vi "02guarda_archivo.vi"(0 "file path nvo":path, 1 "Mediciones":T1, 2 "Mapas Eeprom":T2(array[cluster]), 4 "Equipo nº":i32=30 caption="Eq. nº" min=25 max=100 step=5) -> (5 "error out":errorcluster)   [LabVIEW 2010]
uses:
  <vilib>/Utility/file.llb/Write To Spreadsheet File (string).vi
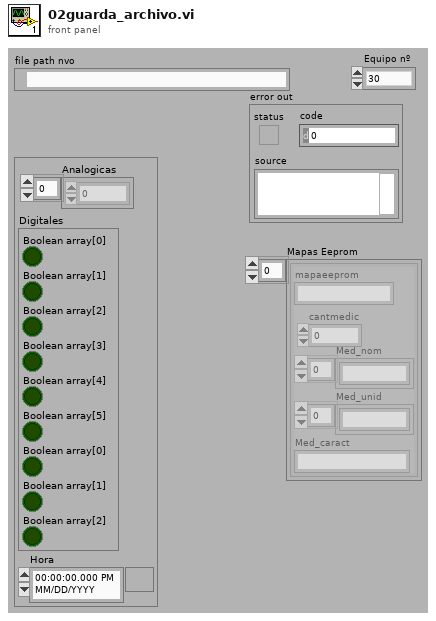
[diagram p1: front panel]
types:
  T1 = cluster{"Analogicas":dbl[], "Digitales":cluster{"Boolean array[0]":bool, "Boolean array[1]":bool, "Boolean array[2]":bool, "Boolean array[3]":bool, "Boolean array[4]":bool, "Boolean array[5]":bool, "Boolean array[0]":bool, "Boolean array[1]":bool, "Boolean array[2]":bool}, "Hora":timestamp}
  T2 = cluster{"mapaeeprom":string, "cantmedic":u8, "Med_nom":string[], "Med_unid":string[], "Med_caract":string}[]
  T3 = enum16{"open", "replace", "create", "open or create", "replace or create", "replace or create with confirmation"}
  T4 = cluster{"Boolean array[0]":bool, "Boolean array[1]":bool, "Boolean array[2]":bool, "Boolean array[3]":bool, "Boolean array[4]":bool, "Boolean array[5]":bool, "Boolean array[0]":bool, "Boolean array[1]":bool, "Boolean array[2]":bool}
  T5 = cluster{"mapaeeprom":string, "cantmedic":u8, "Med_nom":string[], "Med_unid":string[], "Med_caract":string}
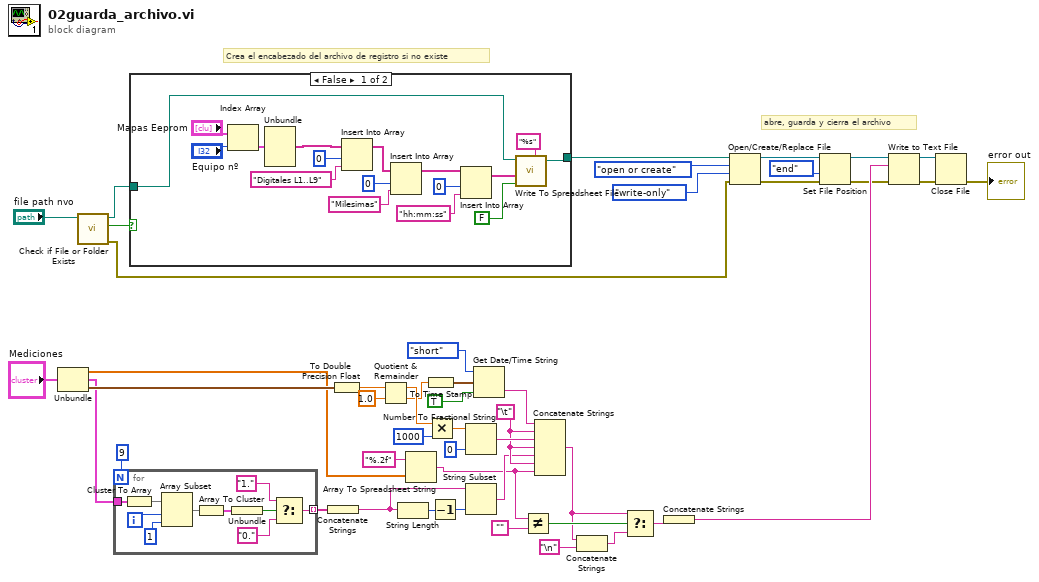
[diagram p0: block diagram]
diagram:
  w26 = "\t"
  # "abre, guarda y cierra el archivo"
  # "Crea el encabezado del archivo de registro si no existe"
  n1 = Unbundle("Mediciones") -> ("Analogicas"=w17:dbl[], "Digitales"=w18:T4, "Hora"=w19:timestamp)
  n2 = call <vilib>:"Check if File or Folder Exists.vi"("path"="file path nvo") -> ("error out"=w1:errorcluster, "file or folder exists?"=w4:bool, "dup path"=w3:path)  [unwired: 8 in]
  n3 = for {
    N: 9 -> [_]
    tunnel: w18 -> [w57]
    tunnel: [w50] -> w24 mode=indexing
    i -> [w52]
    n4 = Cluster To Array(cluster=w57) -> (array=w56:bool[])
    n5 = Array Subset(array=w56, index=w52, length=1) -> (w55:bool[])
    n6 = Array To Cluster(array=w55) -> (cluster=w54:cluster{"[0]":bool})
    n7 = Unbundle(w54) -> ("[0]"=w51:bool)
    n8 = Select(t="1.", s=w51, f="0.") -> (s? t:f=w50:string)
  }
  n9 = case shown="False" w4 {
    tunnel: w3 -> [w63 w75]
    tunnel: [w62 w75] -> w7
    frame False {
      n10 = Index Array(array="Mapas Eeprom", index="Equipo nº") -> (element=w61:T5)
      n11 = Unbundle(w61) -> ("Med_nom"=w58:string[])  [unwired: 4 out]
      n12 = Insert Into Array(array=w58, index=0, new element="Digitales L1..L9" ("new element/subarray")) -> (w71:string[])
      n13 = Insert Into Array(array=w71, index=0, new element="Milesimas" ("new element/subarray")) -> (w69:string[])
      n14 = Insert Into Array(array=w69, index=0, new element="hh:mm:ss" ("new element/subarray")) -> (w68:string[])
      n15 = call-poly <vilib>:"Write To Spreadsheet File.vi"("format (%s)"="%s", "append to file? (new file:F)"=FALSE, "1D data"=w68, "file path (dialog if empty)"=w63) -> ("new file path (Not A Path if cancelled)"=w62:path)  [unwired: 2 in, 2 out]
    }
    frame True {
    }
  }
  n16 = Concatenate Strings(w24) -> (w20:string)
  n17 = To Double Precision Float(number=w19) -> (double precision float=w23:dbl)
  n18 = Quotient & Remainder(x=w23, y=1.0) -> (x-y*floor(x/y)=w32:dbl, floor(x/y)=w27:dbl)
  n19 = String Length(string=w20) -> (length=w22:i32)
  n20 = Array To Spreadsheet String(array=w17, 3:"%.2f" ("format string")) -> (spreadsheet string=w11:string)  [unwired: 1 out]
  n21 = To Time Stamp(1:w27) -> (0:w30:timestamp)
  n22 = Multiply(x=w32, y=1000 ("index")) -> (x*y=w36:dbl)
  n23 = Decrement(x=w22) -> (x-1=w21:i32)
  n24 = Number To Fractional String(number=w36, precision (6)=i16 0) -> (F-format string=w35:string)  [unwired: 2 out]
  n25 = String Subset(string=w20, length (rest)=w21) -> (substring=w16:string)  [unwired: 1 out]
  n26 = Get Date/Time String(date format (0)=enum16{"short", "long", "abbreviated"}."short", seconds (now)=w30, want seconds? (F)=TRUE) -> (time string=w34:string)  [unwired: 1 out]
  n27 = Not Equal?(x=w11, y="") -> (x != y?=w15:bool)
  n28 = Concatenate Strings(w34, w26, w35, w26, w16, w26, w11) -> (w14:string)
  n29 = Concatenate Strings(w14, "\n") -> (w13:string)
  n30 = Select(t=w14, s=w15, f=w13) -> (s? t:f=w42:string)
  n31 = Concatenate Strings(w42) -> (w41:string)
  n32 = Open/Create/Replace File(file path (use dialog)=w7, error in=w1, operation (0:open)=T3."open or create", access (0:read/write)=enum16{"read/write", "read-only", "write-only"}."write-only") -> (refnum out=w47:refnum<file>, error out=w39:errorcluster)  [unwired: 3 out]
  n33 = Set File Position(refnum=w47, from (0:start)=enum16{"start", "end", "current"}."end", error in=w39) -> (refnum out=w43:refnum<file>, error out=w8:errorcluster)  [unwired: 1 out]
  n34 = Write to Text File(file (use dialog)=w43, text=w41, error in=w8) -> (refnum out=w45:refnum<file>, error out=w44:errorcluster)  [unwired: 2 out]
  n35 = Close File(refnum=w45, error in=w44) -> (error out=→"error out":errorcluster)  [unwired: 1 out]
